vi "计算所有paticle在新坐标系坐标.vi"(9 "原点":cluster{dbl, dbl}, 10 "Paticle影像坐标":cluster{dbl, dbl}[](array[cluster]), 11 "角度":dbl) -> (3 "Paticle在产品坐标系坐标":cluster{"X":sgl, "Y":sgl}[](array[cluster]))   [LabVIEW 2014]
uses:
  <vilib>/Analysis/coordinate.llb/2D Cartesian Coordinate Rotation (Scalar).vi
  <vilib>/Analysis/NI_AALPro.lvlib
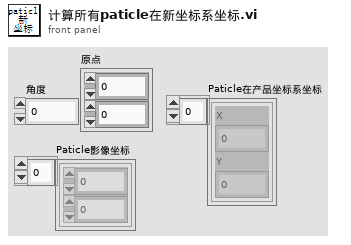
[diagram p1: front panel]
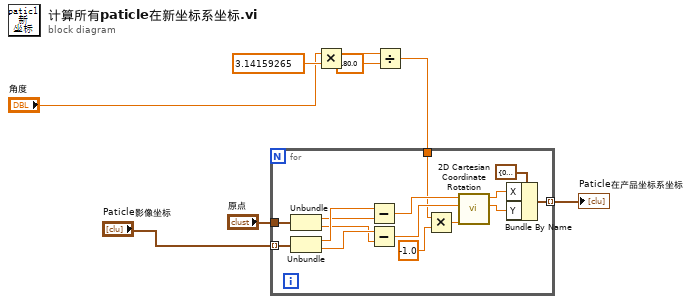
[diagram p0: block diagram]
diagram:
  n1 = Multiply(x="角度", y=3.14159265) -> (x*y=w6:dbl)
  n2 = Divide(x=w6, y=180.0) -> (x/y=w3:dbl)
  n3 = for {
    tunnel: "Paticle影像坐标" -> [w14] mode=indexing
    tunnel: "原点" -> [w11]
    tunnel: w3 -> [w17]
    tunnel: [w21] -> w7 mode=indexing
    n4 = Unbundle(w11) -> (w10:dbl, w9:dbl)
    n5 = Unbundle(w14) -> (w13:dbl, w12:dbl)
    n6 = Subtract(x=w13, y=w10) -> (x-y=w20:dbl)
    n7 = Subtract(x=w12, y=w9) -> (x-y=w19:dbl)
    n8 = Multiply(x=w17, y=-1.0) -> (x*y=w18:dbl)
    n9 = call-poly <vilib>:"2D Cartesian Coordinate Rotation.vi"("theta"=w18, "y"=w19, "x"=w20) -> ("y out"=w22:dbl, "x out"=w23:dbl)  [unwired: 6 in, 1 out]
    n10 = Bundle By Name(cluster=cluster{"X":sgl, "Y":sgl} {"X"=0.0, "Y"=0.0} ("Point2 (Pixels)"), "X"=w23, "Y"=w22) -> (w21:cluster{"X":sgl, "Y":sgl})
  }
  "Paticle在产品坐标系坐标" <- w7
